vi "PH_PILS.get Status of GUI referenced PSU Tags.vi"(1 "PP Tag":T1(array[cluster]), 3 "Tagname":string, 5 "error in":errorcluster) -> (14 "Slider Ref":refnum<vi>, 15 "Head Ref":refnum<vi>, 16 "GUI Ref":refnum<vi>, 17 "Status":i32, 18 "index of element":i32, 19 "error out":errorcluster)   [LabVIEW 2014, in "PH_PILS.lvlib"]
doc: "This VI gets status, array position and GUI ref of the referenced PSU tagname out of the array where the name is set to be the GUI ref."
uses:
  PH_PILS.lvlib
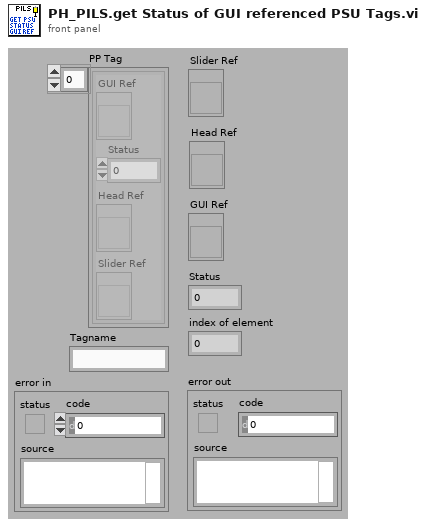
[diagram p1: front panel]
types:
  T1 = cluster{"GUI Ref":refnum<vi>, "Status":i32, "Head Ref":refnum<vi>, "Slider Ref":refnum<vi>}[]
  T2 = cluster{"GUI Ref":refnum<vi>, "Status":i32, "Head Ref":refnum<vi>, "Slider Ref":refnum<vi>}
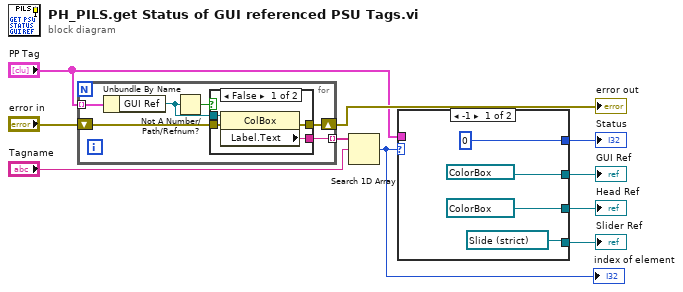
[diagram p0: block diagram]
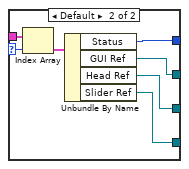
[diagram p2: hidden frame]
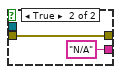
[diagram p3: hidden frame]
diagram:
  n1 = for {
    tunnel: "PP Tag" -> [w16] mode=indexing
    shift-right: [w12] -> w7
    shift-left: "error in" -> [w15]
    tunnel: [w11] -> w5 mode=indexing
    n2 = Unbundle By Name(w16) -> ("GUI Ref"=w13:refnum<vi>)
    n3 = Not A Number/Path/Refnum?(number/path/refnum=w13) -> (NaN/Path/Refnum?=w14:bool)
    n4 = case shown="False" w14 {
      tunnel: w13 -> [w20 _]
      tunnel: w15 -> [w19 w22]
      tunnel: [w18 w22] -> w12
      tunnel: [w17 "N/A" ("Label.Text")] -> w11
      frame False {
        n5 = property class="ColBox"(reference=w20, error in=w19) -> (error out=w18:errorcluster, "Label.Text"=w17:string)  [unwired: 1 out]
      }
      frame True {
      }
    }
  }
  "error out" <- w7
  n6 = Search 1D Array(1D array=w5, element="Tagname") -> (index of element=w9:i32)  [unwired: 1 in]
  "index of element" <- w9
  n7 = case shown="-1" w9 {
    selector: w9 -> [_ w31]
    tunnel: "PP Tag" -> [_ w33]
    tunnel: [0 ("Status") w30] -> w10
    tunnel: [refnum<vi> refnum ("GUI Ref") w29] -> w4
    tunnel: [refnum<vi> refnum ("Head Ref") w28] -> w3
    tunnel: [refnum<vi> refnum ("Slider Ref") w27] -> w1
    frame -1 {
    }
    frame Default {
      n8 = Index Array(array=w33, index=w31) -> (element=w32:T2)
      n9 = Unbundle By Name(w32) -> ("Status"=w30:i32, "GUI Ref"=w29:refnum<vi>, "Head Ref"=w28:refnum<vi>, "Slider Ref"=w27:refnum<vi>)
    }
  }
  "Status" <- w10
  "GUI Ref" <- w4
  "Head Ref" <- w3
  "Slider Ref" <- w1
